vi "PRBS_Generator.vi"(2 "Output Proportion":dbl=1.0, 3 "Repetitions":dbl=2.0) -> (0 "Size":i32, 1 "PRBS Output":dbl)   [LabVIEW 2020]
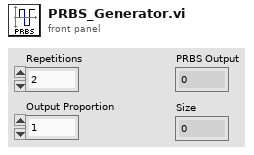
[diagram p1: front panel]
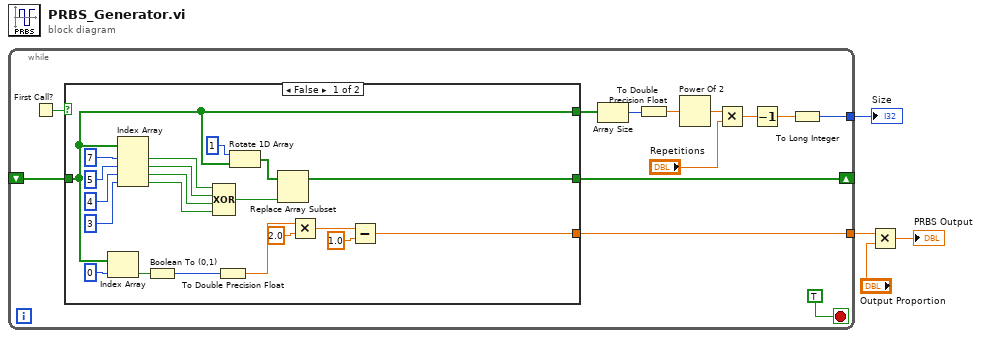
[diagram p0: block diagram]
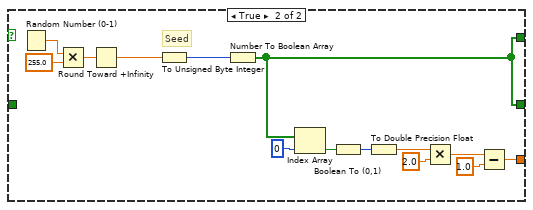
[diagram p2: hidden frame]
diagram:
  n1 = while {
    shift-right: [w16] -> _
    shift-left: _ -> [w15]
    tunnel: [w13] -> w4
    tunnel: [w7] -> w1
    stop <- TRUE stop-if-true
    n2 = First Call?() -> (First Call?: T/F=w17:bool)
    n3 = case shown="False" w17 {
      tunnel: [w21 w39] -> w16
      tunnel: w15 -> [w18 _]
      tunnel: [w19 w40] -> w13
      tunnel: [w18 w39] -> w8
      frame False {
        n4 = Index Array(array=w18, index=0) -> (element=w35:bool)
        n5 = Index Array(array=w18, index #1=7 ("index"), index #2=5 ("index"), index #3=4 ("index"), index #4=3 ("index")) -> (element #1=w29:bool, element #2=w30:bool, element #3=w31:bool, element #4=w32:bool)
        n6 = Boolean To (0,1)(Boolean=w35) -> (0, 1=w36:i16)
        n7 = Compound Arithmetic op=XOR(w29, w30, w31, w32) -> (w33:bool)
        n8 = To Double Precision Float(number=w36) -> (double precision float=w37:dbl)
        n9 = Rotate 1D Array(1:w18, 2:1 ("n")) -> (0:w34:bool[])
        n10 = Replace Array Subset(array=w34, new element=w33) -> (w21:bool[])  [unwired: 1 in]
        n11 = Multiply(x=w37, y=2.0) -> (x*y=w38:dbl)
        n12 = Subtract(x=w38, y=1.0) -> (x-y=w19:dbl)
      }
      frame True {
        # "Seed"
        n13 = Random Number (0-1)() -> (number: 0 to 1=w50:dbl)
        n14 = Multiply(x=w50, y=255.0) -> (x*y=w49:dbl)
        n15 = Round Toward +Infinity(x=w49) -> (ceil(x): smallest int >= x=w51:dbl)
        n16 = To Unsigned Byte Integer(number=w51) -> (unsigned 8bit integer=w52:u8)
        n17 = Number To Boolean Array(number=w52) -> (Boolean array=w39:bool[])
        n18 = Index Array(array=w39, index=0) -> (element=w44:bool)
        n19 = Boolean To (0,1)(Boolean=w44) -> (0, 1=w45:i16)
        n20 = To Double Precision Float(number=w45) -> (double precision float=w46:dbl)
        n21 = Multiply(x=w46, y=2.0) -> (x*y=w47:dbl)
        n22 = Subtract(x=w47, y=1.0) -> (x-y=w40:dbl)
      }
    }
    n23 = Array Size(array=w8) -> (size(s)=w10:i32)
    n24 = To Double Precision Float(number=w10) -> (double precision float=w9:dbl)
    n25 = Power Of 2(x=w9) -> (2^x=w11:dbl)
    n26 = Multiply(x=w11, y="Repetitions") -> (x*y=w12:dbl)
    n27 = Decrement(x=w12) -> (x-1=w6:dbl)
    n28 = To Long Integer(number=w6) -> (32bit integer=w7:i32)
  }
  "Size" <- w1
  n29 = Multiply(x=w4, y="Output Proportion") -> (x*y=→"PRBS Output":dbl)
